vi "AlazarGetBoardRevision.vi"(0 "Handle":u64, 11 "error in (no error)":errorcluster) -> (4 "Handle":u64, 6 "Major Version":u8, 8 "Minor Version":u8, 10 "Return Code":u32, 15 "error out":errorcluster)   [LabVIEW 2018]
doc: "Get the PCB hadware revision level of a digitizer board."
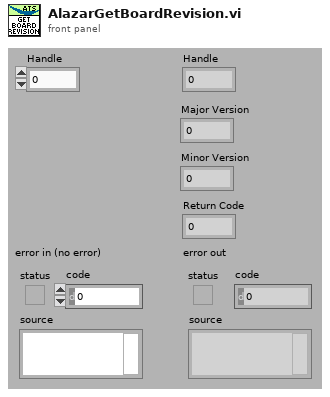
[diagram p1: front panel]
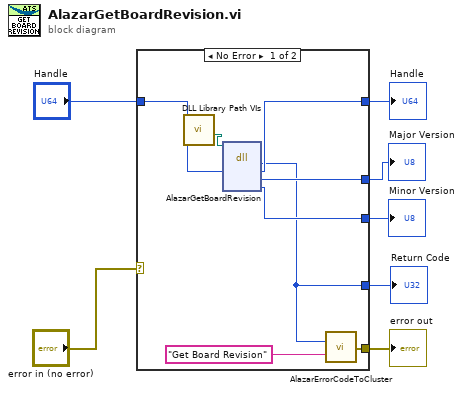
[diagram p0: block diagram]
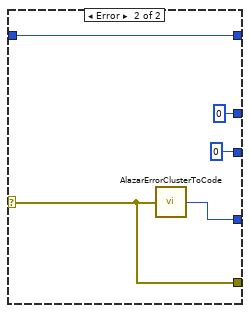
[diagram p2: hidden frame]
diagram:
  n1 = case shown="No Error" "error in (no error)" {
    selector: "error in (no error)" -> [_ w20]
    tunnel: [w11 w20] -> w6
    tunnel: [w10 w19] -> w5
    tunnel: "Handle" -> [w15 w18]
    tunnel: [w14 w18] -> w3
    tunnel: [w13 0] -> w2
    tunnel: [w12 0] -> w1
    frame No Error {
      n2 = call "DLL Library Path VIs.vi"() -> ("Alazar"=w8:path)  [unwired: 9 in, 2 out]
      n3 = dll-call lib="C:/Project/SerialSectOCT - FFT GPU/SerialSectOCT/Labview Software/DLL/ATSApi.dll" fn="AlazarGetBoardRevision"(path in=w8, "handle"=w15) -> ("return type"=w10:u32, "handle"=w14:u64, "majorVersion"=w13:u8, "minorVersion"=w12:u8)  [unwired: 4 in, 2 out]
      n4 = call "AlazarErrorCodeToCluster.vi"("Message"="Get Board Revision", "Error Code"=w10) -> ("error out"=w11:errorcluster)
    }
    frame Error {
      n5 = call "AlazarErrorClusterToCode.vi"("error in (no error)"=w20) -> ("Error Code"=w19:u32)
    }
  }
  "Handle" <- w3
  "error out" <- w6
  "Return Code" <- w5
  "Major Version" <- w2
  "Minor Version" <- w1
